vi "Config GUI - Add To Project.vi"(8 "error in":errorcluster, 11 "GUI Objects":T1) -> (0 "error out":errorcluster, 3 "References of In-Memory Projects":refnum<vi>[](array[refnum]))   [LabVIEW 2021]
doc: "Configures the GUI objects that play a part in the functionality that adds a newly created VI or CTL to an in-memory project."
uses:
  GUI Objects.ctl
  <vilib>/Utility/miscctls.llb/LVFontTypeDef.ctl
panel:
  out "In-Memory Projects":string[](array[string])
  # "Development\ncontrols/indicators useful for development and testing, but which are not outputs of the VI"
  # "Input\nInputs to the VI"
  # "Output\nOutputs of the VI"
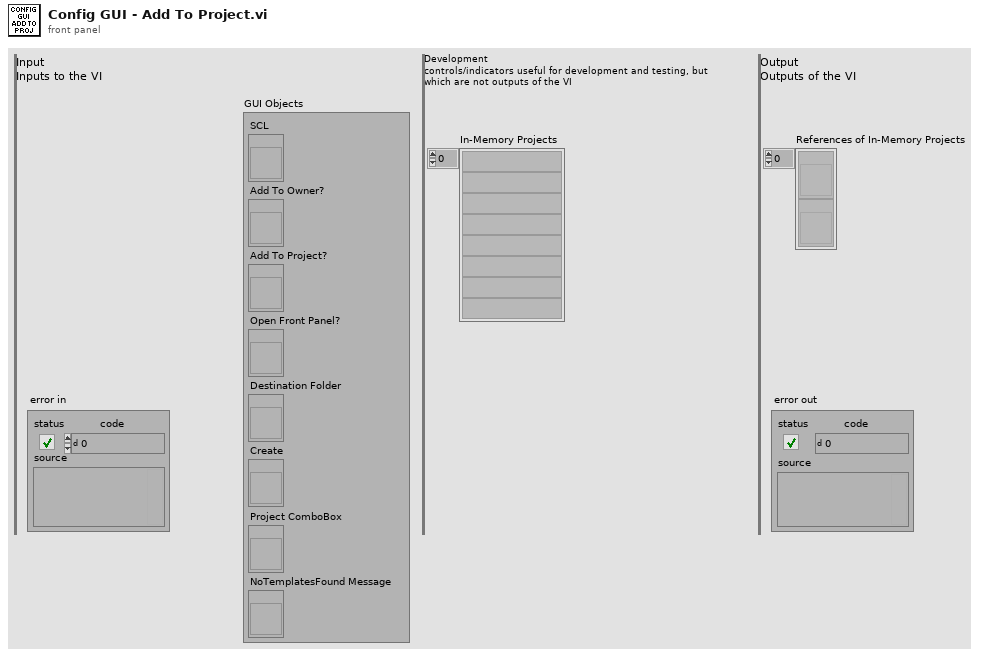
[diagram p1: front panel]
types:
  T1 = typedef "GUI Objects.ctl" = cluster{"SCL":refnum<vi>, "Add To Owner?":refnum<vi>, "Add To Project?":refnum<vi>, "Open Front Panel?":refnum<vi>, "Destination Folder":refnum<vi>, "Create":refnum<vi>, "Project ComboBox":refnum<vi>, "NoTemplatesFound Message":refnum<vi>}
  T2 = typedef "LVFontTypeDef.ctl" = cluster{"Font Name":string, "Size":u16, "Bold":bool, "Italic":bool, "Underline":bool, "Strikeout":bool, "Color":u32}
  T3 = enum8{"Enabled", "Disabled", "Disabled and Grayed Out"}
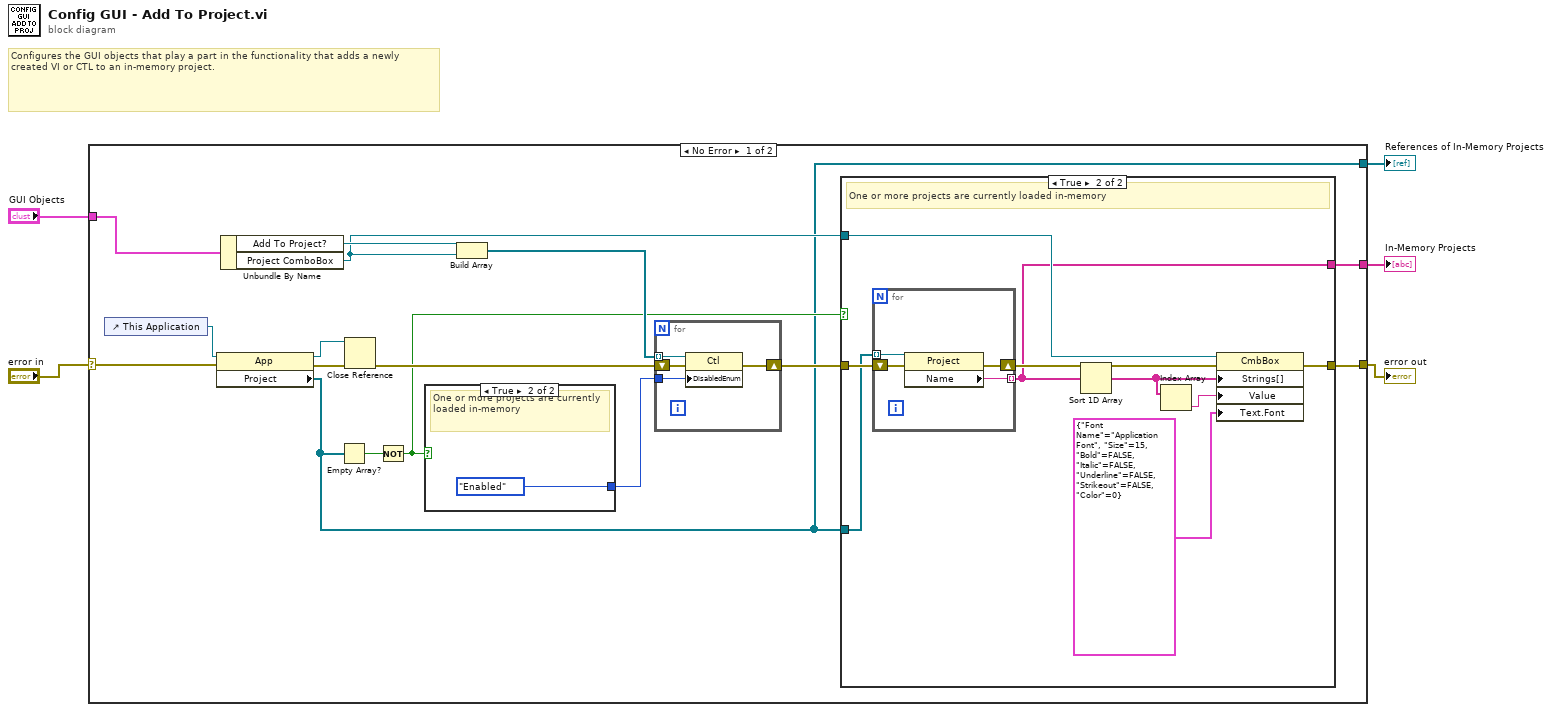
[diagram p0: block diagram]
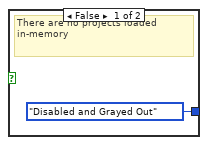
[diagram p3: hidden frame]
diagram:
  # "Configures the GUI objects that play a part in the functionality that adds a newly created VI or CTL to an in-memory project."
  n1 = case shown="No Error" "error in" {
    selector: "error in" -> [w16 w42]
    tunnel: [w10 w42] -> w4
    tunnel: "GUI Objects" -> [w20 _]
    tunnel: [w8 _] -> w2
    tunnel: [w6 _] -> w1
    frame No Error {
      n2 = control-ref of="This Application"() -> (w14:refnum<vi>)
      n3 = property class="App"(reference=w14, error in=w16) -> (reference out=w12:refnum<vi>, error out=w15:errorcluster, "Project"=w6:refnum<vi>[])
      n4 = Unbundle By Name(w20) -> ("Add To Project?"=w19:refnum<vi>, "Project ComboBox"=w9:refnum<vi>)
      n5 = Empty Array?(array=w6) -> (empty?=w11:bool)
      n6 = Close Reference(reference=w12, error in (no error)=w15) -> (error out=w13:errorcluster)
      n7 = Not(x=w11) -> (.not. x?=w7:bool)
      n8 = case shown="True" w7 {
        tunnel: [T3."Disabled and Grayed Out" ("Disabled") T3."Enabled" ("Disabled")] -> w17
        frame False {
          # "There are no projects loaded in-memory"
        }
        frame True {
          # "One or more projects are currently loaded in-memory"
        }
      }
      n9 = Build Array(w19, w9) -> (w18:refnum<vi>[])
      n10 = for {
        shift-right: [w40] -> w21
        shift-left: w13 -> [w41]
        tunnel: w18 -> [w39] mode=indexing
        tunnel: w17 -> [w38]
        n11 = property class="Ctl"(reference=w39, error in=w41, "DisabledEnum"=w38) -> (error out=w40:errorcluster)  [unwired: 1 out]
      }
      n12 = case shown="True" w7 {
        tunnel: w21 -> [w22 w31]
        tunnel: w6 -> [_ w29]
        tunnel: [w22 w28] -> w10
        tunnel: w9 -> [_ w27]
        tunnel: [_ w24] -> w8
        frame False {
          # "There are no projects loaded in-memory"
        }
        frame True {
          # "One or more projects are currently loaded in-memory"
          n13 = for {
            shift-right: [w34] -> w30
            shift-left: w31 -> [w35]
            tunnel: w29 -> [w33] mode=indexing
            tunnel: [w32] -> w24 mode=indexing
            n14 = property class="Project"(reference=w33, error in=w35) -> (error out=w34:errorcluster, "Name"=w32:string)  [unwired: 1 out]
          }
          n15 = Sort 1D Array(array=w24) -> (sorted array=w26:string[])
          n16 = Index Array(array=w26) -> (element=w25:string)  [unwired: 1 in]
          n17 = property class="CmbBox"(reference=w27, error in=w30, "Strings[]"=w26, "Value"=w25, "Text.Font"=T2 {"Font Name"="Application Font", "Size"=15, "Bold"=FALSE, "Italic"=FALSE, "Underline"=FALSE, "Strikeout"=FALSE, "Color"=0}) -> (error out=w28:errorcluster)  [unwired: 1 out]
        }
      }
    }
    frame Error {
    }
  }
  "error out" <- w4
  "In-Memory Projects" <- w2
  "References of In-Memory Projects" <- w1
